vi "test Get RX Mappables.vi"(11 "Test Case In":refnum<class "Test PDO Mapping.lvclass">) -> (0 "error out":errorcluster, 3 "Test Case Out":refnum<class "Test PDO Mapping.lvclass">)   [LabVIEW 2020, in "Test PDO Mapping.lvclass"]
uses:
  Test PDO Mapping.lvclass
  C:/Program Files/National Instruments/LabVIEW 2026/vi.lib/Astemes/LUnit/Test Case.lvclass
  EDS-File-Viewer/source/Electronic Datasheet/Electronic Datasheet.lvclass/Electronic Datasheet.ctl
  <vilib>/Astemes/LUnit/Test Case.lvclass/Test Case.ctl
  4993e8ee-a06a-463a-9684-69129f64d5ce.vi
  EDS-File-Viewer/source/Electronic Datasheet/Electronic Datasheet.lvclass
  source/CANopen.lvlib
  source/Typedefs/Data Type.ctl
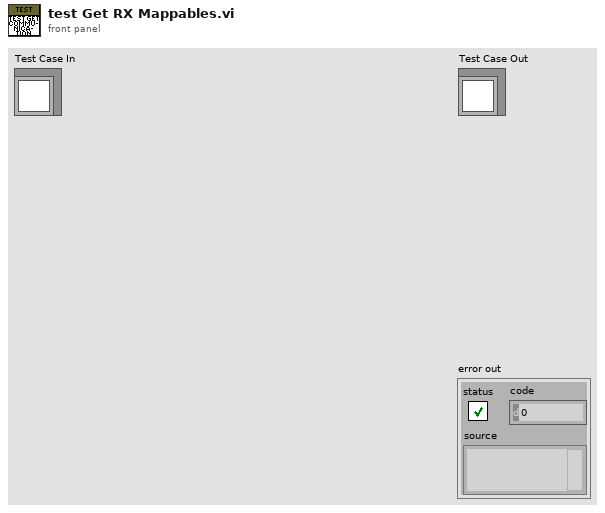
[diagram p1: front panel]
types:
  T1 = typedef "CANopen.lvlib/Data Type.ctl" = u16
  T2 = cluster{"Index":u16, "Sub Index":u8, "Name":string, "Data Type":T1}[]
diagram:
  n1 = Current VI's Path() -> (path=w13:path)
  n2 = Build Path(base path=w13, name or relative path=path "../test.eds") -> (appended path=w10:path)
  n3 = Write to Text File(file (use dialog)=w10, text="[OptionalObjects]\nSupportedObjects=3\n1=0x1F80\n2=0x6402\n3=0x6410\n\n[1F80]\nParameterName=NMTStartup\nObjectType=0x7\nDataType=0x0007\nAccessType=rw\nPDOMapping=0\n\n[6402]\nParameterName=Read Analogue Input 32-Bit\nObjectType=0x8\nSubNumber=21\n\n[6402sub0]\nParameterName=Number of Elements\nObjectType=0x7\nDataType=0x0005\nAccessType=ro\nDefaultValue=20\n\n[6402sub1]\nParameterName=AnalogueInput32[1]\nObjectType=0x7\nDataType=0x0004\nAccessType=rwr\nPDOMapping=1\n\n[6402sub2]\nParameterName=AnalogueInput32[2]\nObjectType=0x7\nDataType=0x0004\nAccessType=rwr\nPDOMapping=1\n\n[6402sub3]\nParameterName=AnalogueInput32[3]\nObjectType=0x7\nDataType=0x0004\nAccessType=rwr\nPDOMapping=1\n\n[6402sub4]\nParameterName=AnalogueInput32[4]\nObjectType=0x7\nDataType=0x0004\nAccessType=rwr\nPDOMapping=1\n\n[6402sub5]\nParameterName=AnalogueInput32[5]\nObjectType=0x7\nDataType=0x0004\nAccessType=rwr\nPDOMapping=1\n\n[6402sub6]\nParameterName=AnalogueInput32[6]\nObjectType=0x7\nDataType=0x0004\nAccessType=rwr\nPDOMapping=1\n\n[6402sub7]\nParameterName=AnalogueInput32[7]\nObjectType=0x7\nDataType=0x0004\nAccessType=rwr\nPDOMapping=1\n\n[6402sub8]\nParameterName=AnalogueInput32[8]\nObjectType=0x7\nDataType=0x0004\nAccessType=rwr\nPDOMapping=1\n\n[6402sub9]\nParameterName=AnalogueInput32[9]\nObjectType=0x7\nDataType=0x0004\nAccessType=rwr\nPDOMapping=1\n\n[6402subA]\nParameterName=AnalogueInput32[10]\nObjectType=0x7\nDataType=0x0004\nAccessType=rwr\nPDOMapping=1\n\n[6402subB]\nParameterName=AnalogueInput32[11]\nObjectType=0x7\nDataType=0x0004\nAccessType=rwr\nPDOMapping=1\n\n[6402subC]\nParameterName=AnalogueInput32[12]\nObjectType=0x7\nDataType=0x0004\nAccessType=rwr\nPDOMapping=1\n\n[6402subD]\nParameterName=AnalogueInput32[13]\nObjectType=0x7\nDataType=0x0004\nAccessType=rwr\nPDOMapping=1\n\n[6402subE]\nParameterName=AnalogueInput32[14]\nObjectType=0x7\nDataType=0x0004\nAccessType=rwr\nPDOMapping=1\n\n[6402subF]\nParameterName=AnalogueInput32[15]\nObjectType=0x7\nDataType=0x0004\nAccessType=rwr\nPDOMapping=1\n\n[6402sub10]\nParameterName=AnalogueInput32[16]\nObjectType=0x7\nDataType=0x0004\nAccessType=rwr\nPDOMapping=1\n\n[6402sub11]\nParameterName=AnalogueInput32[17]\nObjectType=0x7\nDataType=0x0004\nAccessType=rwr\nPDOMapping=1\n\n[6402sub12]\nParameterName=AnalogueInput32[18]\nObjectType=0x7\nDataType=0x0004\nAccessType=rwr\nPDOMapping=1\n\n[6402sub13]\nParameterName=AnalogueInput32[19]\nObjectType=0x7\nDataType=0x0004\nAccessType=rwr\nPDOMapping=1\n\n[6402sub14]\nParameterName=AnalogueInput32[20]\nObjectType=0x7\nDataType=0x0004\nAccessType=rwr\nPDOMapping=1\n\n[6410]\nParameterName=Write Analogue Output 8-Bit\nObjectType=0x8\nSubNumber=21\n\n[6410sub0]\nParameterName=Number of Elements\nObjectType=0x7\nDataType=0x0005\nAccessType=ro\nDefaultValue=20\n\n[6410sub1]\nParameterName=AnalogueOutput8[1]\nObjectType=0x7\nDataType=0x0002\nAccessType=rww\nPDOMapping=1\n\n[6410sub2]\nParameterName=AnalogueOutput8[2]\nObjectType=0x7\nDataType=0x0002\nAccessType=rww\nPDOMapping=1\n\n[6410sub3]\nParameterName=AnalogueOutput8[3]\nObjectType=0x7\nDataType=0x0002\nAccessType=rww\nPDOMapping=1\n\n[6410sub4]\nParameterName=AnalogueOutput8[4]\nObjectType=0x7\nDataType=0x0002\nAccessType=rww\nPDOMapping=1\n\n[6410sub5]\nParameterName=AnalogueOutput8[5]\nObjectType=0x7\nDataType=0x0002\nAccessType=rww\nPDOMapping=1\n\n[6410sub6]\nParameterName=AnalogueOutput8[6]\nObjectType=0x7\nDataType=0x0002\nAccessType=rww\nPDOMapping=1\n\n[6410sub7]\nParameterName=AnalogueOutput8[7]\nObjectType=0x7\nDataType=0x0002\nAccessType=rww\nPDOMapping=1\n\n[6410sub8]\nParameterName=AnalogueOutput8[8]\nObjectType=0x7\nDataType=0x0002\nAccessType=rww\nPDOMapping=1\n\n[6410sub9]\nParameterName=AnalogueOutput8[9]\nObjectType=0x7\nDataType=0x0002\nAccessType=rww\nPDOMapping=1\n\n[6410subA]\nParameterName=AnalogueOutput8[10]\nObjectType=0x7\nDataType=0x0002\nAccessType=rww\nPDOMapping=1\n\n[6410subB]\nParameterName=AnalogueOutput8[11]\nObjectType=0x7\nDataType=0x0002\nAccessType=rww\nPDOMapping=1\n\n[6410subC]\nParameterName=AnalogueOutput8[12]\nObjectType=0x7\nDataType=0x0002\nAccessType=rww\nPDOMapping=1\n\n[6410subD]\nParameterName=AnalogueOutput8[13]\nObjectType=0x7\nDataType=0x0002\nAccessType=rww\nPDOMapping=1\n\n[6410subE]\nParameterName=AnalogueOutput8[14]\nObjectType=0x7\nDataType=0x0002\nAccessType=rww\nPDOMapping=1\n\n[6410subF]\nParameterName=AnalogueOutput8[15]\nObjectType=0x7\nDataType=0x0002\nAccessType=rww\nPDOMapping=1\n\n[6410sub10]\nParameterName=AnalogueOutput8[16]\nObjectType=0x7\nDataType=0x0002\nAccessType=rww\nPDOMapping=1\n\n[6410sub11]\nParameterName=AnalogueOutput8[17]\nObjectType=0x7\nDataType=0x0002\nAccessType=rww\nPDOMapping=1\n\n[6410sub12]\nParameterName=AnalogueOutput8[18]\nObjectType=0x7\nDataType=0x0002\nAccessType=rww\nPDOMapping=1\n\n[6410sub13]\nParameterName=AnalogueOutput8[19]\nObjectType=0x7\nDataType=0x0002\nAccessType=rww\nPDOMapping=1\n\n[6410sub14]\nParameterName=AnalogueOutput8[20]\nObjectType=0x7\nDataType=0x0002\nAccessType=rww\nPDOMapping=1") -> (error out=w9:errorcluster)  [unwired: 2 in, 2 out]
  n4 = call "Import.vi"("error in"=w9, "EDS File Path"=w10) -> ("error out"=w8:errorcluster, "Electronic Datasheet"=w6:refnum<class "Electronic Datasheet.lvclass">)  [unwired: 8 in]
  n5 = call "Get Object Dictionary.vi"("error in"=w8, "Electronic Datasheet in"=w6) -> ("error out"=w7:errorcluster, "Obj Dict"=w5:refnum<class "Object Dictionary.lvclass">)  [unwired: 7 in, 1 out]
  n6 = call "Get PDO Mappables.vi"("error in"=w7, "Type"=enum16{"RX", "TX"}."RX", "Object Dictionary in"=w5) -> ("error out"=w4:errorcluster, "PDO Mappables"=w2:T2)  [unwired: 6 in, 1 out]
  n7 = call "Pass If Equal.vim"("error in (no error)"=w4, "Actual"=w2, "Expected"=T2 [{"Index"=25616, "Sub Index"=1, "Name"="AnalogueOutput8[1]", "Data Type"=2}, {"Index"=25616, "Sub Index"=2, "Name"="AnalogueOutput8[2]", "Data Type"=2}, {"Index"=25616, "Sub Index"=3, "Name"="AnalogueOutput8[3]", "Data Type"=2}, {"Index"=25616, "Sub Index"=4, "Name"="AnalogueOutput8[4]", "Data Type"=2}, {"Index"=25616, "Sub Index"=5, "Name"="AnalogueOutput8[5]", "Data Type"=2}, {"Index"=25616, "Sub Index"=6, "Name"="AnalogueOutput8[6]", "Data Type"=2}, {"Index"=25616, "Sub Index"=7, "Name"="AnalogueOutput8[7]", "Data Type"=2}, {"Index"=25616, "Sub Index"=8, "Name"="AnalogueOutput8[8]", "Data Type"=2}, {"Index"=25616, "Sub Index"=9, "Name"="AnalogueOutput8[9]", "Data Type"=2}, {"Index"=25616, "Sub Index"=10, "Name"="AnalogueOutput8[10]", "Data Type"=2}, {"Index"=25616, "Sub Index"=11, "Name"="AnalogueOutput8[11]", "Data Type"=2}, {"Index"=25616, "Sub Index"=12, "Name"="AnalogueOutput8[12]", "Data Type"=2}, {"Index"=25616, "Sub Index"=13, "Name"="AnalogueOutput8[13]", "Data Type"=2}, {"Index"=25616, "Sub Index"=14, "Name"="AnalogueOutput8[14]", "Data Type"=2}, {"Index"=25616, "Sub Index"=15, "Name"="AnalogueOutput8[15]", "Data Type"=2}, {"Index"=25616, "Sub Index"=16, "Name"="AnalogueOutput8[16]", "Data Type"=2}, {"Index"=25616, "Sub Index"=17, "Name"="AnalogueOutput8[17]", "Data Type"=2}, {"Index"=25616, "Sub Index"=18, "Name"="AnalogueOutput8[18]", "Data Type"=2}, {"Index"=25616, "Sub Index"=19, "Name"="AnalogueOutput8[19]", "Data Type"=2}, {"Index"=25616, "Sub Index"=20, "Name"="AnalogueOutput8[20]", "Data Type"=2}] ("PDO Mappables"), "LUnit Test Case In"="Test Case In") -> ("error out"=→"error out":errorcluster, "LUnit Test Case Out"=→"Test Case Out":refnum<class "Test PDO Mapping.lvclass">)  [unwired: 6 in]
